vi "SR830 set time constant.vi"(8 "error in (no error)":errorcluster, 10 "Tau":u16(ring) items=["10 us", "30 us", "100 us", "300 us", "1 ms", "3 ms", "10 ms", "30 ms", "100 ms", "300 ms", "1 s", "3 s", "10 s", "30 s", "100 s", "300 s", "1 ks", "3 ks", "10 ks", "30 ks"], 11 "VISA resource name":refnum<visa-resource-name>) -> (0 "error out":errorcluster, 3 "VISA resource name out":refnum<visa-resource-name>)   [LabVIEW 2009, in "SR830.lvlib"]
doc: "Sets the current reference mode (internal or external) of the lock-in amplifier."
uses:
  SR830.lvlib
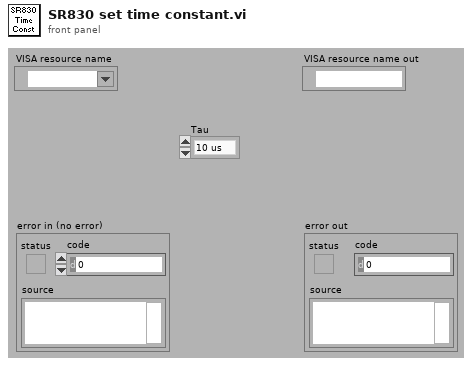
[diagram p1: front panel]
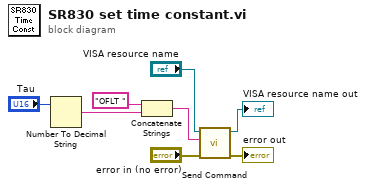
[diagram p0: block diagram]
diagram:
  n1 = Number To Decimal String(number="Tau") -> (decimal integer string=w7:string)  [unwired: 1 in]
  n2 = Concatenate Strings("OFLT " ("write buffer"), w7) -> (w5:string)
  n3 = call "Send Command.vi"("error in (no error)"="error in (no error)", "write buffer"=w5, "VISA resource name"="VISA resource name") -> ("error out"=→"error out":errorcluster, "VISA resource name out"=→"VISA resource name out":refnum<visa-resource-name>)  [unwired: 7 in]
